vi "FGVStop.vi"(7 "Set? (False)":bool, 8 "Error In":errorcluster[](array[cluster]), 11 "Value to Set (False)":bool) -> (0 "Error Out":errorcluster[](array[cluster]), 3 "Value":bool)   [LabVIEW 2018, in "Visualization.lvlib" / "VisualizeBase.lvclass"]
doc: "Functional global variable that can be used to stop implement a remote stop for various visualization vis."
uses:
  VisualizeBase.lvclass
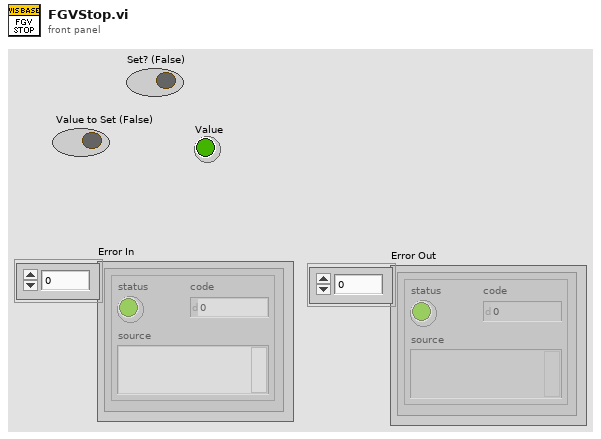
[diagram p1: front panel]
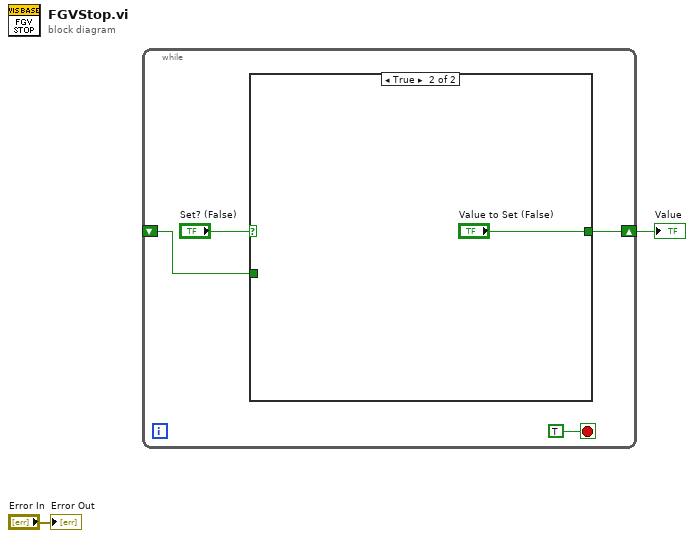
[diagram p0: block diagram]
diagram:
  n1 = while {
    shift-right: [w5] -> w2
    shift-left: _ -> [w3]
    stop <- TRUE stop-if-true
    n2 = case shown="True" "Set? (False)" {
      tunnel: [w7 "Value to Set (False)"] -> w5
      tunnel: w3 -> [w7 _]
      frame False {
      }
      frame True {
      }
    }
  }
  "Value" <- w2
  "Error Out" <- "Error In"
